vi "FM_RX.vi"() -> ()   [LabVIEW 2013]
uses:
  <vilib>/sound2/lvsound2.llb/Sound Data Format.ctl
  <vilib>/sound2/lvsound2.llb/Sound Output Write (DBL Single).vi
  <vilib>/Analysis/2dsp.llb/Rational Resample (single channel, DBL).vi
  <vilib>/Waveform/WDTFileIO.llb/Read Waveform from File.vi
  <vilib>/Analysis/NI_AALPro.lvlib
  <userlib>/FMDemodRTLSDR_DLL/FMDemodRTLSDR_DLL.lvlib
panel:
  out "Waveform":waveform(dbl)(graph)
  out "error out":errorcluster
  in  "file path (dialog if empty)":path=path "D:/Data_IQIQ"
  out "error out":errorcluster
  in  "sound format":T1={"sample rate (S/s)"=44100.0, "number of channels"=1, "bits per sample"=16}
  in  "stop":bool
  in  "IQ rate":u32=286650
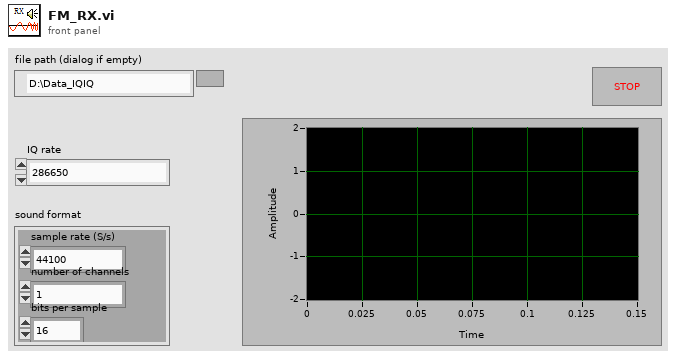
[diagram p1: front panel]
types:
  T1 = typedef "Sound Data Format.ctl" = cluster{"sample rate (S/s)":dbl, "number of channels":i32, "bits per sample":i32}
  T2 = typedef "Sound Output Task ID.ctl" = u32
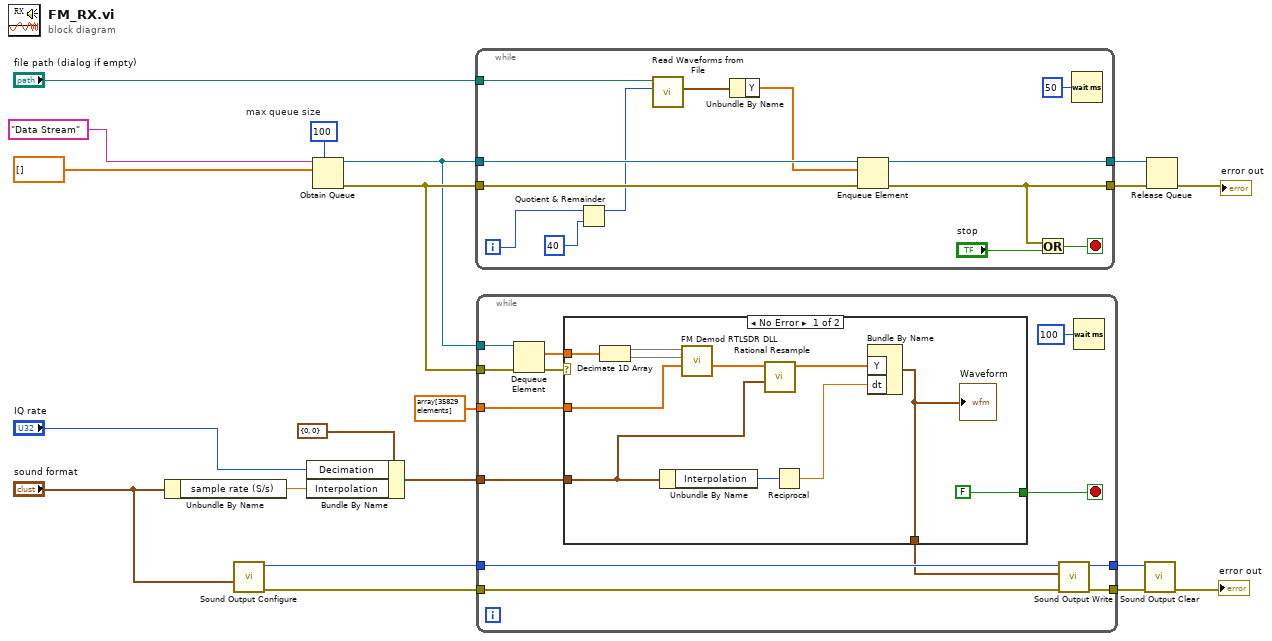
[diagram p0: block diagram]
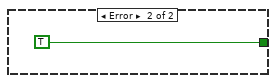
[diagram p2: hidden frame]
diagram:
  w4 = 100  # max queue size
  n1 = Unbundle By Name("sound format") -> ("sample rate (S/s)"=w7:dbl)
  n2 = call <vilib>:"Sound Output Configure.vi"("sound format"="sound format") -> ("error out"=w2:errorcluster, "task ID"=w17:T2)  [unwired: 9 in]
  n3 = Bundle By Name(cluster=cluster{"Interpolation":i32, "Decimation":i32} {"Interpolation"=0, "Decimation"=0}, "Decimation"="IQ rate", "Interpolation"=w7) -> (w10:cluster{"Interpolation":i32, "Decimation":i32})
  n4 = Obtain Queue(max queue size (-1, unlimited)=w4, name (unnamed)="Data Stream", element data type=dbl[] [] ("buf 2")) -> (queue out=w8:refnum<queue>, error out=w9:errorcluster)  [unwired: 2 in, 1 out]
  n5 = while {
    tunnel: w8 -> [w33]
    tunnel: [w22] -> w13
    tunnel: w9 -> [w32]
    tunnel: [w31] -> w12
    tunnel: "file path (dialog if empty)" -> [w28]
    i -> [w25]
    stop <- w29 stop-if-true
    n6 = Quotient & Remainder(x=w25, y=40) -> (x-y*floor(x/y)=w23:i32)  [unwired: 1 out]
    n7 = call-poly <vilib>:"Read Waveforms from File.vi"("offset (records:0)"=w23, "file path (dialog if empty)"=w28) -> ("first waveform in record"=w27:waveform(dbl))  [unwired: 4 in, 3 out]
    n8 = Unbundle By Name(w27) -> ("Y"=w26:dbl[])
    n9 = Enqueue Element(queue=w33, element=w26, error in (no error)=w32) -> (queue out=w22:refnum<queue>, error out=w31:errorcluster)  [unwired: 1 in, 1 out]
    n10 = Or(x=w31, y="stop") -> (x .or. y?=w29:bool)
    n11 = Wait (ms)(milliseconds to wait=u32 50) -> ()  [unwired: 1 out]
  }
  n12 = while {
    tunnel: w17 -> [w41]
    tunnel: [w45] -> w16
    tunnel: [w44] -> w15
    tunnel: w2 -> [w46]
    tunnel: w8 -> [w43]
    tunnel: w10 -> [w37]
    tunnel: w9 -> [w42]
    tunnel: dbl[] array[35829 elements] ("Baseband") -> [w39]
    stop <- w35 stop-if-true
    n13 = Dequeue Element(queue=w43, error in (no error)=w42) -> (element=w40:dbl[], error out=w36:errorcluster)  [unwired: 1 in, 2 out]
    n14 = case shown="No Error" w36 {
      tunnel: w40 -> [w56 _]
      tunnel: w39 -> [w52 _]
      tunnel: [w47 _] -> w38
      tunnel: w37 -> [w51 _]
      tunnel: [FALSE TRUE] -> w35
      frame No Error {
        n15 = Decimate 1D Array(w56) -> (w55:dbl[], w54:dbl[])
        n16 = Unbundle By Name(w51) -> ("Interpolation"=w50:i32)
        n17 = call <userlib>:"FM Demod RTLSDR DLL.vi"("Baseband"=w52, "QSamples"=w54, "ISamples"=w55) -> ("Baseband out"=w53:dbl[])  [unwired: 7 in, 1 out]
        n18 = call-poly <vilib>:"Rational Resample.vi"("resample factor"=w51, "X"=w53) -> ("Y"=w57:dbl[])  [unwired: 7 in, 2 out]
        n19 = Reciprocal(x=w50) -> (1/x=w49:dbl)
        n20 = Bundle By Name ("Build Waveform")("Y"=w57, "dt"=w49) -> (w47:waveform(dbl))  [unwired: 1 in]
        "Waveform" <- w47
      }
      frame Error {
      }
    }
    n21 = call-poly <vilib>:"Sound Output Write.vi"("error in (no error)"=w46, "data"=w38, "task ID"=w41) -> ("error out"=w44:errorcluster, "task ID out"=w45:T2)  [unwired: 7 in]
    n22 = Wait (ms)(milliseconds to wait=u32 100) -> ()  [unwired: 1 out]
  }
  n23 = call <vilib>:"Sound Output Clear.vi"("error in (no error)"=w15, "task ID"=w16) -> ("error out"=→"error out":errorcluster)  [unwired: 9 in]
  n24 = Release Queue(queue=w13, error in (no error)=w12) -> (error out=→"error out":errorcluster)  [unwired: 1 in, 2 out]
